vi "resetView.vi"(8 "error in (no error)":errorcluster, 11 "AbstractMultiColumnListBoxAdapter in":refnum<class "AbstractMultiColumnListBoxAdapter.lvclass">) -> (0 "error out":errorcluster, 3 "AbstractMultiColumnListBoxAdapter out":refnum<class "AbstractMultiColumnListBoxAdapter.lvclass">)   [LabVIEW 2020, in "AbstractMultiColumnListBoxAdapter.lvclass"]
uses:
  AbstractMultiColumnListBoxAdapter.lvclass
  <vilib>/Utility/miscctls.llb/LVRowAndColumnUnsignedTypeDef.ctl
  AbstractMultiColumnListBoxAdapter.lvclass/AbstractMultiColumnListBoxAdapter.ctl
  <vilib>/Utility/miscctls.llb/LVRowAndColumnTypeDef.ctl
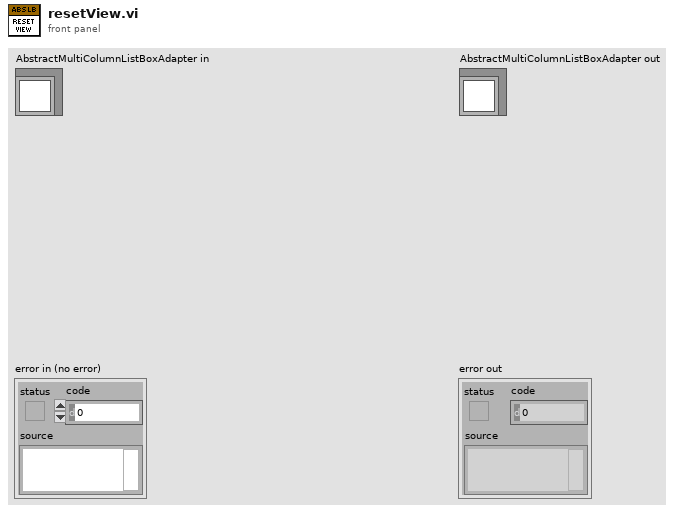
[diagram p1: front panel]
types:
  T1 = typedef "LVRowAndColumnUnsignedTypeDef.ctl" = cluster{"Row":u32, "Column":u32}
  T2 = typedef "LVRowAndColumnTypeDef.ctl" = cluster{"Row":i32, "Column":i32}
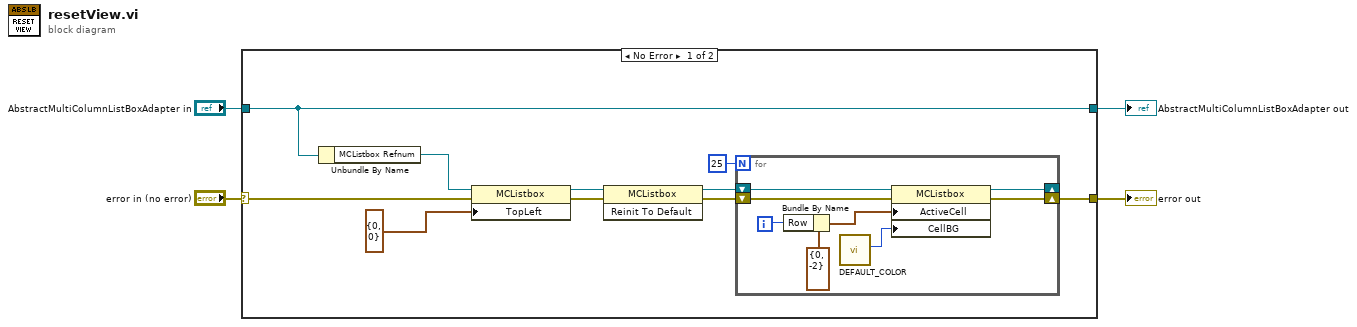
[diagram p0: block diagram]
diagram:
  n1 = case shown="No Error" "error in (no error)" {
    selector: "error in (no error)" -> [w10 w24]
    tunnel: [w5 w24] -> w1
    tunnel: [w14 w23] -> w2
    tunnel: "AbstractMultiColumnListBoxAdapter in" -> [w14 w23]
    frame No Error {
      n2 = Unbundle By Name(w14) -> ("MCListbox Refnum"=w13:refnum<vi>)
      n3 = property class="MCListbox"(reference=w13, error in=w10, "TopLeft"=T1 {"Row"=0, "Column"=0} ("Top Left Visible Cell")) -> (reference out=w12:refnum<vi>, error out=w11:errorcluster)
      n4 = invoke class="MCListbox" method="Reinit To Default"(reference=w12, error in=w11) -> (reference out=w6:refnum<vi>, error out=w7:errorcluster)  [unwired: 1 in, 1 out]
      n5 = for {
        N: 25 -> [_]
        shift-right: [w21] -> _
        shift-left: w6 -> [w22]
        shift-right: [w19] -> w5
        shift-left: w7 -> [w20]
        i -> [w17]
        n6 = Bundle By Name(cluster=T2 {"Row"=0, "Column"=-2} ("Active Cell:Active Cell"), "Row"=w17) -> (w16:T2)
        n7 = call "DEFAULT_COLOR.vi"() -> ("Color Box"=w15:u32)  [unwired: 11 in]
        n8 = property on="Property Node" class="MCListbox"(reference=w22, error in=w20, "ActiveCell"=w16, "CellBG"=w15) -> (reference out=w21:refnum<vi>, error out=w19:errorcluster)
      }
    }
    frame Error {
    }
  }
  "error out" <- w1
  "AbstractMultiColumnListBoxAdapter out" <- w2
